vi "roboRIO v1.0 Timer ISR Worker.vi"(11 "IRQ Number":u8) -> ()   [LabVIEW 2021]
uses:
  <vilib>/myRIO/Common/Instrument Driver Framework/Utilities/typedefs/FPGA Ref Manager Action Enum.ctl
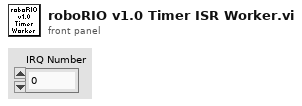
[diagram p1: front panel]
types:
  T1 = typedef "FPGA Ref Manager Action Enum.ctl" = enum16{"Get", "Set", "Reset"}
  T2 = typedef "Generic FPGA Reference.ctl" = refnum<k20>
  T3 = typedef "Callback VI Ref.ctl" = refnum<vi>
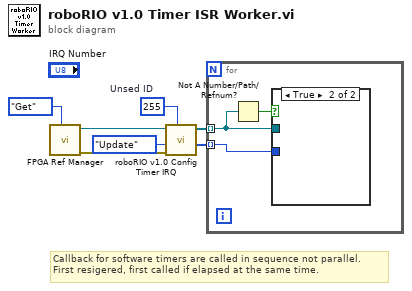
[diagram p0: block diagram]
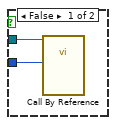
[diagram p2: hidden frame]
diagram:
  w2 = u8 255  # Unsed ID
  # "Callback for software timers are called in sequence not parallel. \nFirst resigered, first called if elapsed at the same time."
  n1 = call <vilib>:"FPGA Ref Manager.vi"("Action"=FPGA_Ref_Manager_Action_Enum."Get") -> ("error out"=w5:errorcluster, "Generic FPGA Reference out"=w6:T2)  [unwired: 8 in]
  n2 = call <vilib>:"roboRIO v1.0 Config Timer IRQ.vi"("Timer ID"=w2, "error in (no error)"=w5, "Action"=enum16{"Add", "Update", "Remove"}."Update", "myRIO FPGA Ref In"=w6) -> ("Timer IDs"=w4:u8[], "Callback VI Refs"=w3:T3[])  [unwired: 5 in, 1 out]
  n3 = for {
    tunnel: w4 -> [w9] mode=indexing
    tunnel: w3 -> [w8] mode=indexing
    n4 = Not A Number/Path/Refnum?(number/path/refnum=w8) -> (NaN/Path/Refnum?=w10:bool)
    n5 = case shown="True" w10 {
      tunnel: w9 -> [w12 _]
      tunnel: w8 -> [w11 _]
      frame False {
        n6 = call-by-ref "?"(reference=w11, "ID"=w12) -> ()  [unwired: 12 in, 2 out]
      }
      frame True {
      }
    }
  }
